vi "Stop Core.vi"(10 "final error code":i32, 11 "InterferometrUI in":refnum<class "InterferometryUI.lvclass">) -> (3 "InterferometrUI out":refnum<class "InterferometryUI.lvclass">)   [LabVIEW 2023, in "InterferometryUI.lvlib" / "InterferometryUI.lvclass"]
doc: "(<B>Filename</B>: Actor Framework.lvlib:Actor.lvclass:Stop Core.vi)\n\nDefines what the actor does before it stops. Use the <B>final error code</B> input to determine whether the actor shut down in response to an error.\n\nBy default, this method passes the Stop message along to all auto-stop nested actors. A descendant class may override this method to define additional behavior, such as shutting down any processes the actor initiated in its override of the Actor Core method."
uses:
  InterferometryUI.lvclass
  <vilib>/ActorFramework/Actor/Actor.lvclass
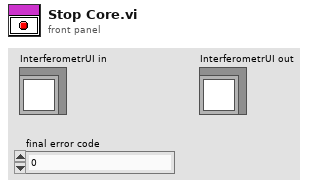
[diagram p1: front panel]
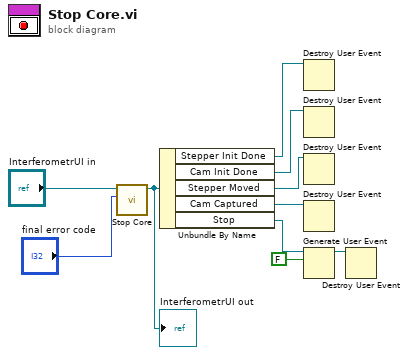
[diagram p0: block diagram]
diagram:
  n1 = call-parent "Stop Core.vi"("final error code"="final error code", "Actor in"="InterferometrUI in") -> ("Actor out"=w2:refnum<class "InterferometryUI.lvclass">)  [unwired: 9 in]
  "InterferometrUI out" <- w2
  n2 = Unbundle By Name(w2) -> ("Stepper Init Done"=w3:refnum<user-event>, "Cam Init Done"=w4:refnum<user-event>, "Stepper Moved"=w5:refnum<user-event>, "Cam Captured"=w6:refnum<user-event>, "Stop"=w8:refnum<user-event>)
  n3 = Destroy User Event(user event=w3) -> ()  [unwired: 1 in, 1 out]
  n4 = Destroy User Event(user event=w4) -> ()  [unwired: 1 in, 1 out]
  n5 = Destroy User Event(user event=w5) -> ()  [unwired: 1 in, 1 out]
  n6 = Destroy User Event(user event=w6) -> ()  [unwired: 1 in, 1 out]
  n7 = Generate User Event(user event=w8, event data cluster=FALSE ("event data")) -> (user event out=w7:refnum<user-event>)  [unwired: 2 in, 1 out]
  n8 = Destroy User Event(user event=w7) -> ()  [unwired: 1 in, 1 out]
